vi "main.vi"() -> ()   [LabVIEW 2014]
uses:
  <vilib>/Math Plots/3D Math Plots/3D Scatter/3D Scatter XCtrl/3D Scatter.xctl
  <vilib>/Utility/miscctls.llb/LV3DPointTypeDef.ctl
  <vilib>/Utility/miscctls.llb/LVRectTypeDef.ctl
  <vilib>/Math Plots/3D Math Plots/3D Scatter/3D Scatter Datatype/Public/Plot Helper (Vector).vi
  Kinect SDK v1.0/Kinect SDK v1.0/Kinect Library/Kinect Library.lvlib
  <vilib>/Math Plots/3D Math Plots/3D Scatter/3D Scatter Datatype/3D Scatter Datatype.lvclass
  <vilib>/picture/3D Picture Control/NI_3D Picture Control.lvlib
panel:
  out "Map Data out":T1(array[cluster])
  in  "Update time":dbl
  in  "Chunk length (voxel)":u8=8
  in  "voxel length (in.)":dbl=8.0 format="%#_13g"
  out "3d map Kbytes":dbl format="%#_3f"
  out "Framerate":dbl
  in  "Kinect FOV (deg)":cluster{"Height":i32, "Width":i32}={"Height"=43, "Width"=57}
  in  "Sensor Yaw angle (deg)":sgl
  in  "Sensor position":cluster{"X":sgl, "Y":sgl, "Z":sgl}={"X"=0.0, "Y"=0.0, "Z"=70.75}
  out "3D view":refnum<class "3D Plot Datatype.lvclass">[](xcontrol)
  in  "New Width":i32=80
  in  "New Height":i32=60
  out "Color Frame":T2(plugin-control)
  in  "Elevation Angle":i32(slide) scale=-27.0..27.0
  out "Depth Frame":T2(plugin-control)
  in  "stop":bool
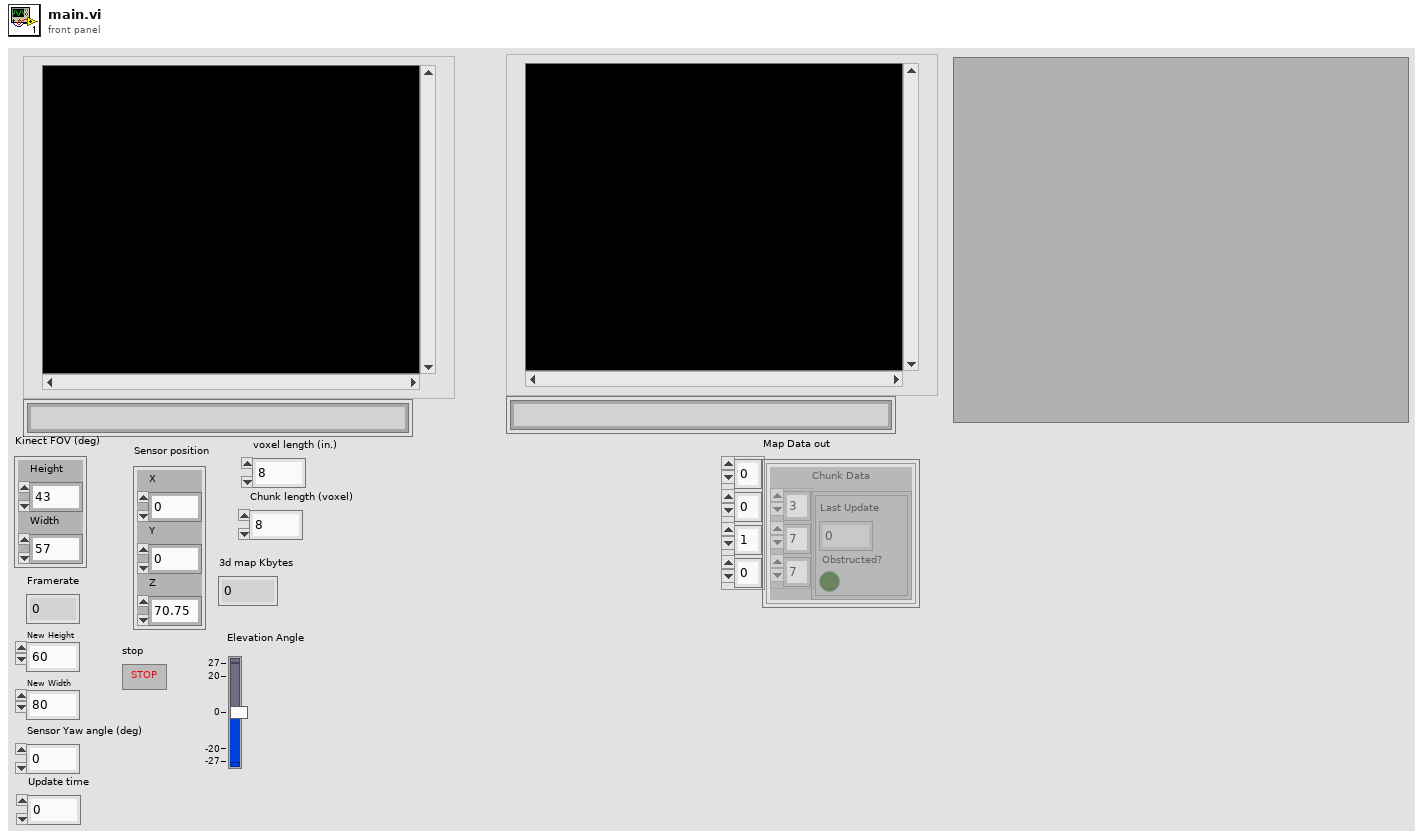
[diagram p1: front panel]
types:
  T1 = cluster{"Chunk Data":cluster{"Last Update":u32, "Obstructed?":bool}[][][]}[][][][]
  T2 = typedef "IMAQ Image.ctl" = refnum<image>
  T3 = typedef "LVRectTypeDef.ctl" = cluster{"Left":i16, "Top":i16, "Right":i16, "Bottom":i16}
  T4 = typedef "LV3DPointTypeDef.ctl" = cluster{"X":sgl, "Y":sgl, "Z":sgl}
  T5 = typedef "Image Type" = u32
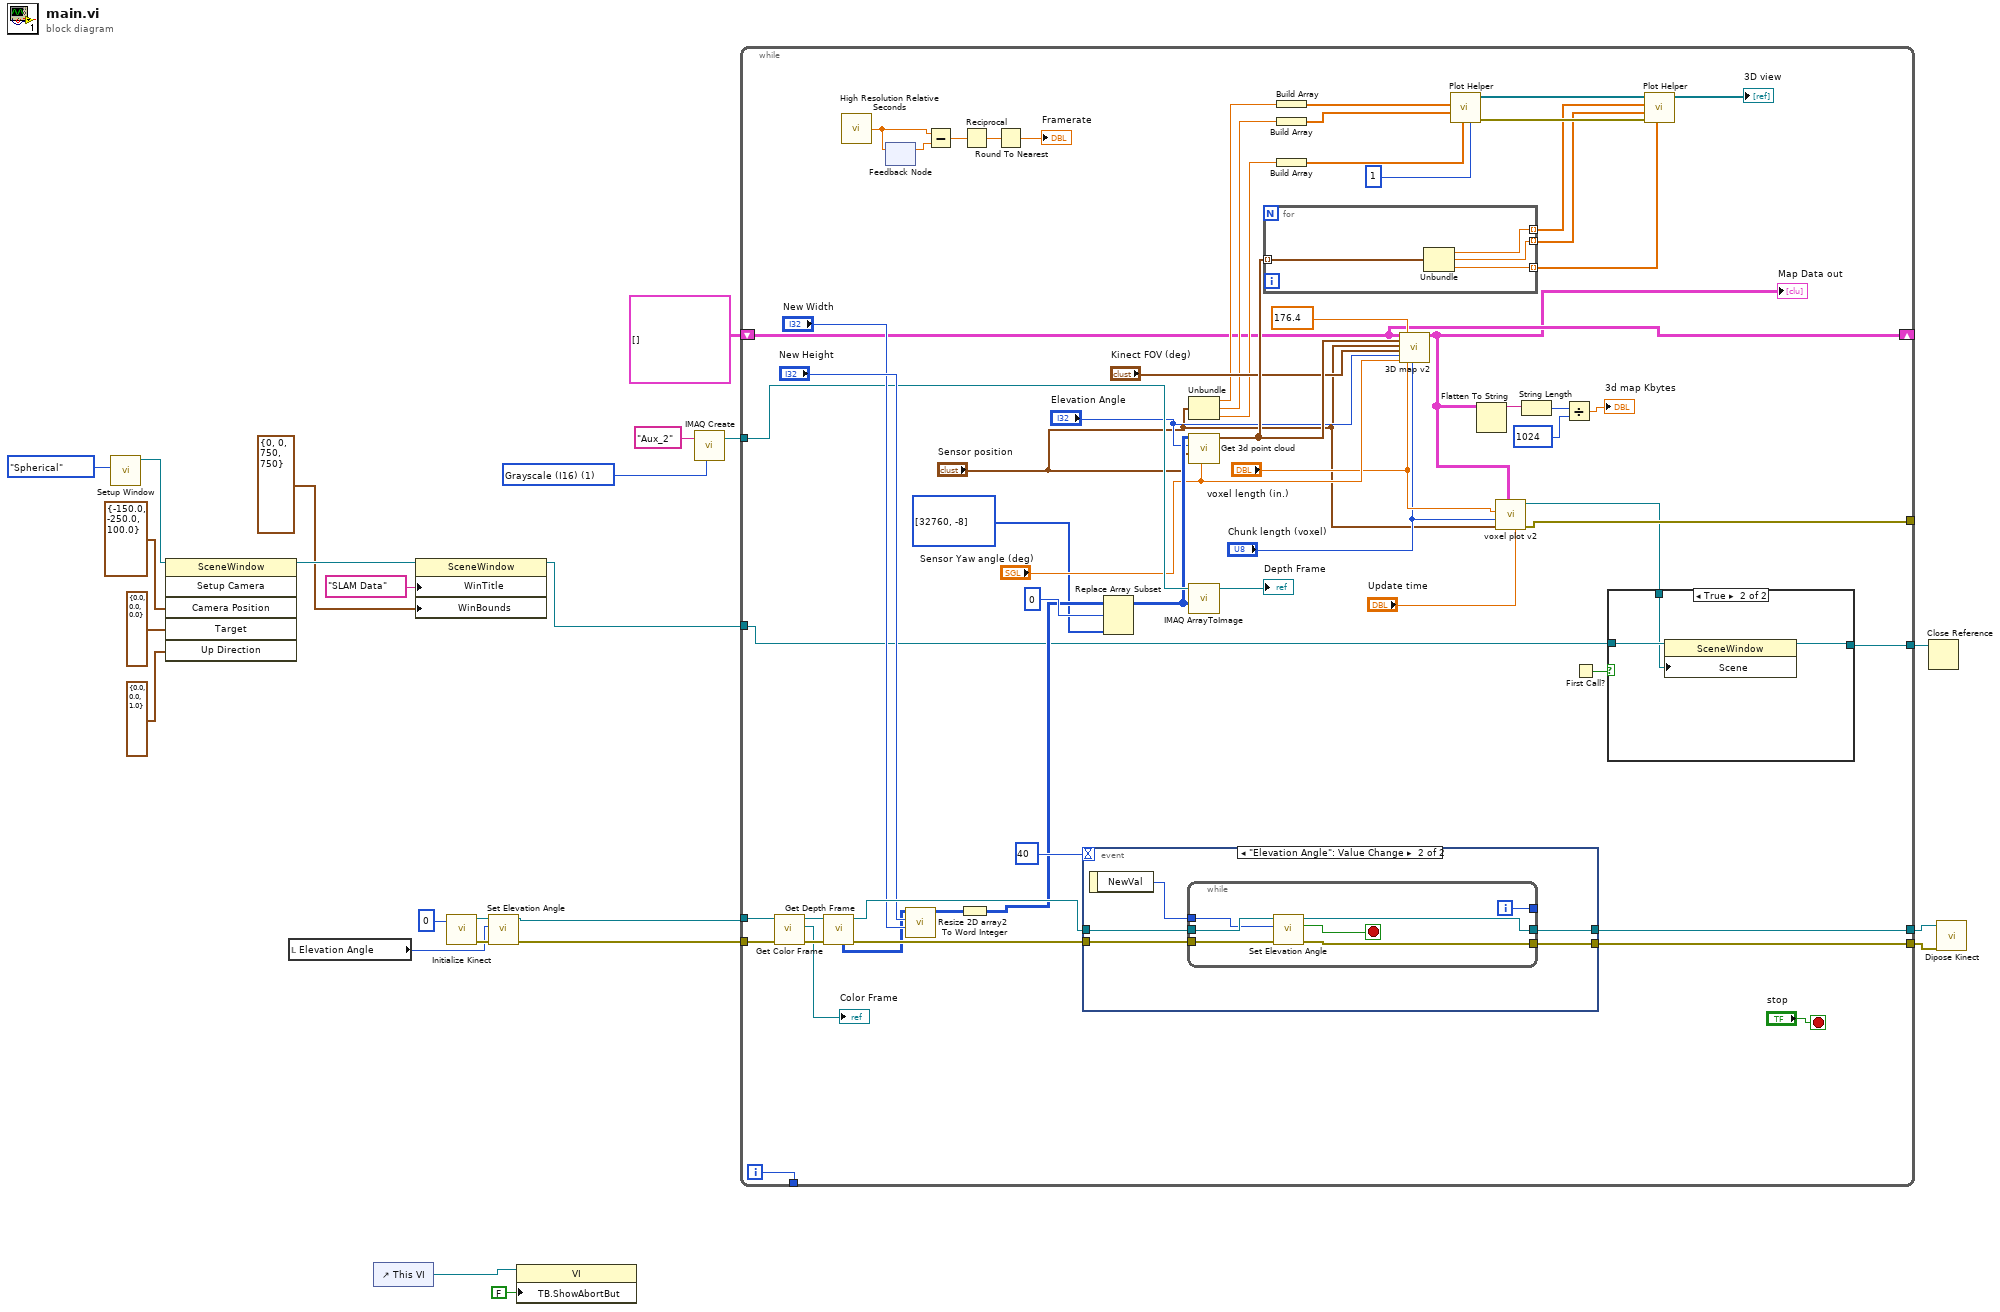
[diagram p0: block diagram]
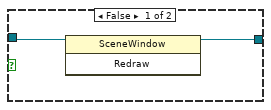
[diagram p2: hidden frame]
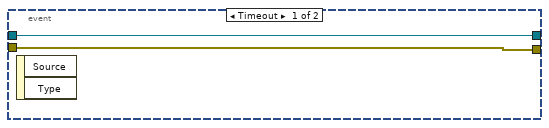
[diagram p3: hidden frame]
diagram:
  w18 = T5 1 items=["Grayscale (U8)", "Grayscale (I16)", "Grayscale (SGL)", "Complex (CSG)", "RGB (U32)", "HSL (U32)", "RGB (U64)", "Grayscale (U16)"] ("Image Type")
  n1 = call <vilib>:"Setup Window.vi"("Camera Controller"=enum16{"None", "Spherical", "Flying"}."Spherical") -> ("New Window Refnum"=w9:refnum<vi>)  [unwired: 9 in, 1 out]
  n2 = invoke class="SceneWindow" method="Setup Camera"(reference=w9, "Camera Position"=T4 {"X"=-150.0, "Y"=-250.0, "Z"=100.0}, "Target"=T4 {"X"=0.0, "Y"=0.0, "Z"=0.0}, "Up Direction"=T4 {"X"=0.0, "Y"=0.0, "Z"=1.0}) -> (reference out=w5:refnum<vi>)  [unwired: 2 in, 5 out]
  n3 = local read "Elevation Angle"() -> (w14:i32)
  n4 = control-ref of="This VI"() -> (w22:refnum<vi>)
  n5 = property class="SceneWindow"(reference=w5, "WinTitle"="SLAM Data" ("Window Title"), "WinBounds"=T3 {"Left"=0, "Top"=0, "Right"=750, "Bottom"=750} ("Window Bounds")) -> (reference out=w2:refnum<vi>)  [unwired: 1 in, 1 out]
  n6 = call "Initialize Kinect.vi"("Kinect Sensor Index"=0 ("ElevationAngle")) -> ("error out"=w17:errorcluster, "Kinect Session out"=w16:refnum<class "Kinect Session.lvclass">)  [unwired: 9 in]
  n7 = call "Set Elevation Angle.vi"("error in (no error)"=w17, "ElevationAngle"=w14, "Kinect Session in"=w16) -> ("error out"=w11:errorcluster, "Kinect Session out"=w12:refnum<class "Kinect Session.lvclass">)  [unwired: 6 in, 1 out]
  n8 = property class="VI"(reference=w22, "TB.ShowAbortBut"=FALSE ("Tool Bar:Show Abort Button")) -> ()  [unwired: 1 in, 2 out]
  n9 = call "IMAQ Create"("Image Name"="Aux_2", "Image Type"=w18) -> ("New Image"=w19:T2)  [unwired: 3 in, 1 out]
  n10 = while {
    tunnel: [w78] -> w24
    tunnel: [w77] -> w23
    tunnel: w19 -> [w69]
    tunnel: w12 -> [w67]
    tunnel: w11 -> [w66]
    shift-right: [w30] -> _
    shift-left: T1 [] ("Map Data out") -> [w30]
    tunnel: [w33] -> _
    tunnel: [w32] -> _
    tunnel: w2 -> [w29]
    tunnel: [w26] -> w1
    i -> [w33]
    stop <- "stop" stop-if-true
    n11 = call "Get Color Frame.vi"("error in (no error)"=w66, "Kinect Session in"=w67) -> ("error out"=w82:errorcluster, "Color Frame"=→"Color Frame":T2, "Kinect Session out"=w83:refnum<class "Kinect Session.lvclass">)  [unwired: 7 in]
    n12 = call "Get Depth Frame.vi"("error in (no error)"=w82, "Kinect Session in"=w83) -> ("error out"=w79:errorcluster, "Kinect Session out"=w80:refnum<class "Kinect Session.lvclass">, "Pixel depth array"=w73:i16[][])  [unwired: 5 in, 2 out]
    n13 = call <vilib>:"High Resolution Relative Seconds.vi"() -> ("relative seconds"=w45:dbl)
    n14 = feedback-in #1(w45) -> ()
    n15 = feedback #1() -> (w44:dbl)  [unwired: 1 in]
    n16 = call "Resize 2D array2.vi"("New Width"="New Width", "New Height"="New Height", "2D Array In"=w73) -> ("Resized Array"=w71:i32[][])  [unwired: 4 in]
    n17 = Subtract(x=w45, y=w44) -> (x-y=w43:dbl)
    n18 = To Word Integer(number=w71) -> (16bit integer=w70:i16[][])
    n19 = Reciprocal(x=w43) -> (1/x=w42:dbl)
    n20 = Round To Nearest(number=w42) -> (nearest integer value=→"Framerate":dbl)
    n21 = event shown="[1] \"Elevation Angle\": Value Change" {
      selector: _ -> [_ _]
      dyn-events: _ -> [_ _]
      timeout: 40 -> [_ _]
      tunnel: w80 -> [w95 w100]
      tunnel: w79 -> [w94 w99]
      tunnel: [w95 w98] -> w78
      tunnel: [w94 w97] -> w77
      event Timeout {
        n22 = event-data() -> ()  [unwired: 1 in, 2 out]
      }
      event "Elevation Angle": Value Change {
        n23 = event-data() -> ("NewVal"=w96:i32)  [unwired: 1 in]
        n24 = while {
          tunnel: w100 -> [w106]
          tunnel: w99 -> [w105]
          tunnel: [w104] -> w98
          tunnel: [w103] -> w97
          tunnel: w96 -> [w102]
          tunnel: [w101] -> _
          i -> [w101]
          stop <- w107 stop-if-true
          n25 = call "Set Elevation Angle.vi"("error in (no error)"=w105, "ElevationAngle"=w102, "Kinect Session in"=w106) -> ("error out"=w103:errorcluster, "Success?"=w107:bool, "Kinect Session out"=w104:refnum<class "Kinect Session.lvclass">)  [unwired: 6 in]
        }
      }
    }
    n26 = Replace Array Subset(array=w70, new element=i16[] [32760, -8], index (row)=i16 0) -> (w64:i16[][])  [unwired: 1 in]
    n27 = Unbundle("Sensor position") -> ("X"=w51:sgl, "Y"=w48:sgl, "Z"=w46:sgl)
    n28 = call "Get 3d point cloud.vi"("Sensor Yaw"="Sensor Yaw angle (deg)", "Sensor position"="Sensor position", "Elevation Angle"="Elevation Angle", "Depth Array"=w64) -> ("Points"=w57:cluster{"Data":sgl, "Data":sgl, "Data":sgl}[])  [unwired: 7 in]
    n29 = call "IMAQ ArrayToImage"("Image Pixels (I16)"=w64, "Image"=w69) -> ("Image Out"=→"Depth Frame":T2)  [unwired: 8 in, 1 out]
    n30 = for {
      tunnel: w57 -> [w93] mode=indexing
      tunnel: [w92] -> w61 mode=indexing
      tunnel: [w91] -> w60 mode=indexing
      tunnel: [w90] -> w59 mode=indexing
      n31 = Unbundle(w93) -> ("Data"=w92:sgl, "Data"=w91:sgl, "Data"=w90:sgl)
    }
    n32 = Build Array(w51) -> (w50:sgl[])
    n33 = Build Array(w48) -> (w49:sgl[])
    n34 = Build Array(w46) -> (w47:sgl[])
    n35 = call "3D map v2.vi"("Map Data in"=w30, "3d Points"=w57, "Sensor position"="Sensor position", "Kinect FOV (deg)"="Kinect FOV (deg)", "Elevation Angle"="Elevation Angle", "Sensor Yaw angle (deg)"="Sensor Yaw angle (deg)", "Max distance"=176.4, "voxel length (in.)"="voxel length (in.)", "Chunk length (voxel)"="Chunk length (voxel)") -> ("Map Data out"=w25:T1)  [unwired: 10 in]
    "Map Data out" <- w25
    n36 = call-poly <vilib>:"Plot Helper.vi"("Plot ID"=1, "z vector"=w47, "y vector"=w49, "x vector"=w50) -> ("error out"=w63:errorcluster, "3D Plot lvclass Array out"=w62:refnum<class "3D Plot Datatype.lvclass">[])  [unwired: 2 in, 4 out]
    n37 = Flatten To String(anything=w25) -> (data string=w40:string)  [unwired: 3 in, 2 out]
    n38 = call "voxel plot v2.vi"("Update time"="Update time", "Map Data In"=w25, "Sensor position"="Sensor position", "Chunk length"="Chunk length (voxel)", "voxel length"="voxel length (in.)") -> ("error out"=w32:errorcluster, "Scene"=w28:refnum<vi>)  [unwired: 3 in]
    n39 = String Length(string=w40) -> (length=w39:i32)
    n40 = Divide(x=w39, y=1024) -> (x/y=→"3d map Kbytes":dbl)
    n41 = First Call?() -> (First Call?: T/F=w27:bool)
    n42 = case shown="True" w27 {
      tunnel: w29 -> [w86 w89]
      tunnel: w28 -> [_ w88]
      tunnel: [w85 w87] -> w26
      frame False {
        n43 = invoke class="SceneWindow" method="Redraw"(reference=w86) -> (reference out=w85:refnum<vi>)  [unwired: 2 in, 2 out]
      }
      frame True {
        n44 = property class="SceneWindow"(reference=w89, "Scene"=w88) -> (reference out=w87:refnum<vi>)  [unwired: 1 in, 1 out]
      }
    }
    n45 = call-poly <vilib>:"Plot Helper.vi"("z vector"=w59, "error in (no error)"=w63, "y vector"=w60, "x vector"=w61, "3D Plot lvclass Array in"=w62) -> ("3D Plot lvclass Array out"=→"3D view":refnum<class "3D Plot Datatype.lvclass">[])  [unwired: 1 in, 5 out]
  }
  n46 = Close Reference(reference=w1) -> ()  [unwired: 1 in, 1 out]
  n47 = call "Dipose Kinect.vi"("error in (no error)"=w23, "Kinect Session in"=w24) -> ()  [unwired: 9 in, 1 out]
